vi "slscswitch Disconnect All Channels.vi"(8 "error in (no error)":errorcluster, 11 "SLSC Switch in":refnum<class "SLSC Switch.lvclass">) -> (0 "error out":errorcluster, 3 "SLSC Switch out":refnum<class "SLSC Switch.lvclass">)   [LabVIEW 2015, in "SLSC Switch.lvclass"]
uses:
  SLSC Switch.lvclass
  SLSC Switch.lvclass/SLSC Switch.ctl
  Route Manager/Route Manager.lvclass
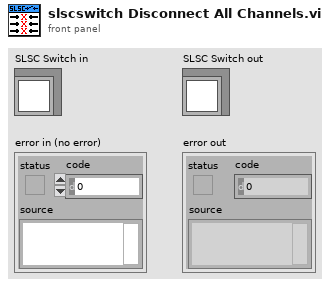
[diagram p1: front panel]
types:
  T1 = typedef "Route Manager.lvclass/Connection.ctl" = cluster{"channel 1":string, "channel 2":string}
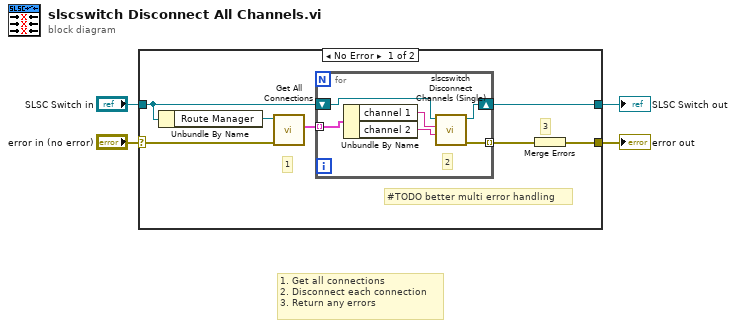
[diagram p0: block diagram]
diagram:
  # "1. Get all connections\n2. Disconnect each connection\n3. Return any errors"
  n1 = case shown="No Error" "error in (no error)" {
    selector: "error in (no error)" -> [w10 w19]
    tunnel: [w5 w19] -> w3
    tunnel: [w8 w18] -> w1
    tunnel: "SLSC Switch in" -> [w9 w18]
    frame No Error {
      # "3"
      # "1"
      # "#TODO better multi error handling"
      n2 = Unbundle By Name(w9) -> ("Route Manager"=w11:refnum<class "Route Manager.lvclass">)
      n3 = call "Get All Connections.vi"("error in (no error)"=w10, "Route Manager in"=w11) -> ("connections"=w7:T1[])  [unwired: 8 in, 1 out]
      n4 = for {
        shift-right: [w16] -> w8
        shift-left: w9 -> [w17]
        tunnel: w7 -> [w15] mode=indexing
        tunnel: [w12] -> w6 mode=indexing
        # "2"
        n5 = Unbundle By Name(w15) -> ("channel 1"=w14:string, "channel 2"=w13:string)
        n6 = call "slscswitch Disconnect Channels (Single).vi"("channel 2"=w13, "channel 1"=w14, "SLSC Switch in"=w17) -> ("error out"=w12:errorcluster, "SLSC Switch out"=w16:refnum<class "SLSC Switch.lvclass">)  [unwired: 7 in]
      }
      n7 = Merge Errors(w6) -> (w5:errorcluster)
    }
    frame Error {
    }
  }
  "error out" <- w3
  "SLSC Switch out" <- w1
